vi "Set ToolTipText.vi"(8 "error in":errorcluster, 10 "ToolTipText":string, 11 "Cell in":refnum<class "Cell.lvclass">) -> (0 "error out":errorcluster, 3 "Cell out":refnum<class "Cell.lvclass">)   [LabVIEW 2024, in "SourceGrid.lvlib" / "Cell.lvclass"]
uses:
  Cell.lvclass
  Cell.lvclass/Cell.ctl
  D:/git/Sourcegrid-LabVIEW/dll/SourceGrid.dll
  dll/SourceGrid.dll
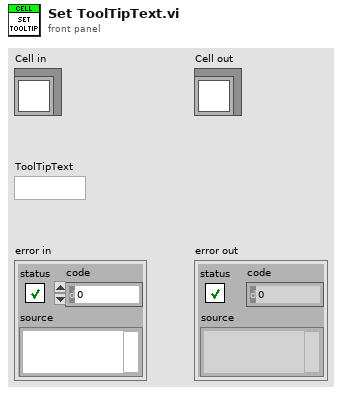
[diagram p1: front panel]
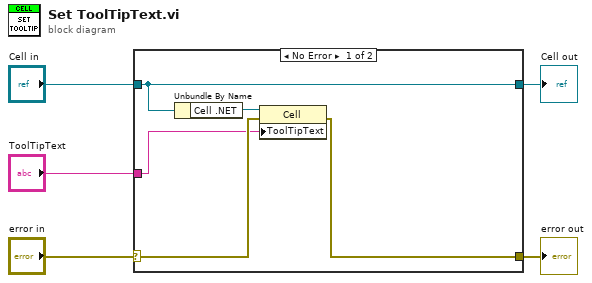
[diagram p0: block diagram]
diagram:
  n1 = case shown="No Error" "error in" {
    selector: "error in" -> [w9 w11]
    tunnel: [w7 w11] -> w4
    tunnel: [w10 w12] -> w2
    tunnel: "Cell in" -> [w10 w12]
    tunnel: "ToolTipText" -> [w6 _]
    frame No Error {
      n2 = Unbundle By Name(w10) -> ("Cell .NET"=w8:refnum<k24>)
      n3 = property class="Cell"(reference=w8, error in=w9, "ToolTipText"=w6) -> (error out=w7:errorcluster)  [unwired: 1 out]
    }
    frame Error {
    }
  }
  "error out" <- w4
  "Cell out" <- w2
